vi "SWI Driver.vi"(5 "SWI Configuration (\"\")":string, 6 "Drv Refnum":T1, 7 "SWI Command":T2, 8 "error in (no error)":errorcluster, 10 "SWI Position In":variant) -> (0 "error out":errorcluster, 1 "SWI Flat Output":string, 2 "SWI Position Out":variant, 4 "dup Drv Refnum":T1)   [LabVIEW 2011]
uses:
  SWI Command.ctl
  SWI Driver Ref.ctl
panel:
  in  "DEBUG?":bool
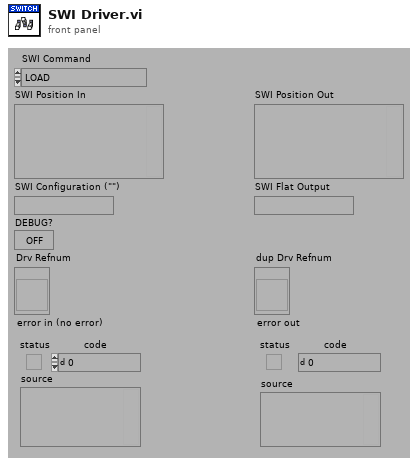
[diagram p1: front panel]
types:
  T1 = typedef "SWI Driver Ref.ctl" = refnum<vi>
  T2 = typedef "SWI Command.ctl" = enum16{"LOAD", "INITIALIZE", "PRESET", "SET STIMULUS", "GET STIMULUS", "GET INFO", "RELEASE", "UNLOAD"}
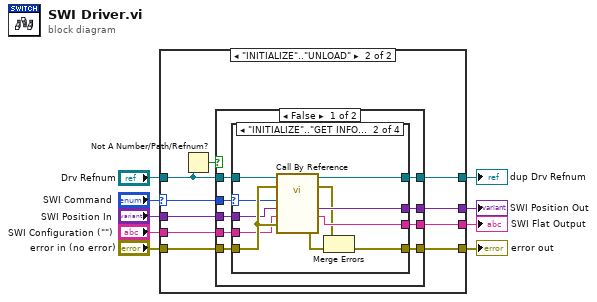
[diagram p0: block diagram]
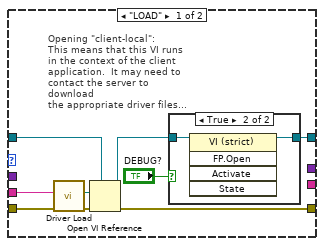
[diagram p2: hidden frame]
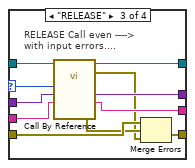
[diagram p5: hidden frame]
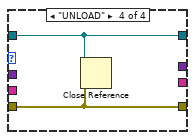
[diagram p6: hidden frame]
diagram:
  n1 = case shown="\"INITIALIZE\"..\"UNLOAD\"" "SWI Command" {
    selector: "SWI Command" -> [_ w24]
    tunnel: "error in (no error)" -> [w18 w31]
    tunnel: "SWI Position In" -> [_ w30]
    tunnel: [_ w29] -> w7
    tunnel: [w17 w28] -> w6
    tunnel: "SWI Configuration (\"\")" -> [w16 w27]
    tunnel: [_ w26] -> w4
    tunnel: [w15 w25] -> w3
    tunnel: "Drv Refnum" -> [w14 w23]
    frame "LOAD" {
      # "Opening \"client-local\":\nThis means that this VI runs\nin the context of the client\napplication.  It may need to\ncontact the server to download\nthe appropriate driver files..."
      n2 = call "Driver Load.vi"("error in (no error)"=w18, "DriverID DriverType (\"\")"=w16) -> ("error out"=w10:errorcluster, "Driver Component Path"=w11:path)  [unwired: 1 in, 7 out]
      n3 = Open VI Reference(type specifier VI Refnum (for type only)=w14, vi path=w11, error in (no error)=w10) -> (vi reference=w13:T1, error out=w17:errorcluster)  [unwired: 3 out]
      n4 = case shown="True" "DEBUG?" {
        tunnel: w13 -> [w19 w21]
        tunnel: [w19 w20] -> w15
        frame False {
        }
        frame True {
          n5 = invoke class="VI (strict)" method="FP.Open"(reference=w21) -> (reference out=w20:T1)  [unwired: 4 in, 4 out]
        }
      }
    }
    frame "INITIALIZE".."UNLOAD" {
      n6 = Not A Number/Path/Refnum?(number/path/refnum=w23) -> (NaN/Path/Refnum?=w22:bool)
      n7 = case shown="False" w22 {
        tunnel: w31 -> [w40 w67]
        tunnel: w30 -> [w39 _]
        tunnel: [w38 _] -> w29
        tunnel: [w37 w67] -> w28
        tunnel: w27 -> [w36 _]
        tunnel: [w35 _] -> w26
        tunnel: [w34 w68] -> w25
        tunnel: w23 -> [w33 w68]
        tunnel: w24 -> [w32 _]
        frame False {
          n8 = case shown="\"INITIALIZE\"..\"GET INFO\"" w32 {
            selector: w32 -> [_ w46 w59 _]
            tunnel: w40 -> [w42 w50 w57 w65]
            tunnel: w39 -> [_ w47 w60 _]
            tunnel: [_ w49 w62 _] -> w38
            tunnel: [w42 w53 w64 w65] -> w37
            tunnel: w36 -> [_ w45 w58 _]
            tunnel: [_ w48 w61 _] -> w35
            tunnel: [w41 w51 w63 w66] -> w34
            tunnel: w33 -> [w41 w52 w54 w66]
            frame "LOAD", Default {
              # "This will not ever run."
            }
            frame "INITIALIZE".."GET INFO" {
              n9 = call-by-ref "?"(reference=w52, error in=w50, "error in (no error)"=w50, "SWI Configuration (\"\")"=w45, "SWI Position In"=w47, "SWI Command"=w46) -> (reference out=w51:T1, error out=w43:errorcluster, 0:"error out"=w44:errorcluster, "SWI Flat Output"=w48:string, "SWI Position Out"=w49:variant)  [unwired: 5 in]
              n10 = Merge Errors(w43, w44) -> (w53:errorcluster)
            }
            frame "RELEASE" {
              # "RELEASE Call even ---->\nwith input errors...."
              n11 = call-by-ref "?"(reference=w54, "SWI Configuration (\"\")"=w58, "SWI Position In"=w60, "SWI Command"=w59) -> (reference out=w63:T1, error out=w55:errorcluster, 0:"error out"=w56:errorcluster, "SWI Flat Output"=w61:string, "SWI Position Out"=w62:variant)  [unwired: 7 in]
              n12 = Merge Errors(w57, w56, w55) -> (w64:errorcluster)
            }
            frame "UNLOAD" {
              n13 = Close Reference(reference=w66, error in (no error)=w65) -> ()  [unwired: 1 out]
            }
          }
        }
        frame True {
          # "If the reference is not valid\nno operation is performed."
        }
      }
    }
  }
  "error out" <- w6
  "SWI Position Out" <- w7
  "SWI Flat Output" <- w4
  "dup Drv Refnum" <- w3
